vi "Project Data InitialS3.vi"(11 "configuration file path":path=path "C:/Users/MyUser/Desktop/新文字文件 - 複製.txt") -> (1 "Step Content":string[][](table), 2 "Retry":i32, 3 "process cluster":cluster{string[], i32[]})   [LabVIEW 2019]
uses:
  <vilib>/Utility/config.llb/Read Key (String).vi
  <vilib>/Utility/config.llb/NI_LVConfig.lvlib
  Ctrl/StationCmdSelect.ctl
  FlowCtrl Class/LineScan/LineScan.lvclass
  Ctrl/MeasureDisplayTab.ctl
  LLB/Commonly VI/Main Glb.vi
  LLB/Commonly VI.lvlib
  Ctrl/Table Save.ctl
  Ctrl/Auto Inspection Station Name2.ctl
  Ctrl/Auto Inspection Data Name.ctl
  Ctrl/S2 Station IO.ctl
panel:
  out "S2 receive":string
  out "Blue Scan2 receive":string
  out "T2 buffer":string
  out "T2 μA":dbl format="%#_6f"
  out "T1 buffer":string
  out "T1 μA":dbl format="%#_6f"
  in  "error in (no error)":errorcluster
  out "Blue Scan receive":string
  out "S1 receive":string
  out "Program receive":string
  out "Initial receive":string
  out "Act Step":i32
  out "retry次數":string[](array[string])
  in  "stop":bool
  out "Boolean":bool=TRUE
  in  "Numeric 3":i32
  out "format receive":string
  out "CurrentCmd":string
  out "Numeric":dbl
  out "LOG":string[][](array[string])
  in  "Enum":T1(ring)=enum."Add"
  in  "Table Control 3":string[][](table)=[["PCBA BARCODE", ""], ["硬體(Tool初始化)", ""], ["company(Tool初始化)", ""], ["耗電流 uA(電流表)", "T"], ["電池負載電壓", "T"], ["晶片ID(Tool FORMAT)", "F"], ["雷雕ID(TOOl scan、藍芽接收器)", "S"], ["Format(Tool FORMAT)", "F"], ["Programe(Tool Programe)", "P"]]
  in  "SN":string
  out "Array 3":cluster{"Table Control":string[][]}[](array[cluster])
  in  "Table Control":string[][](table)=[["PCBA BARCODE", ""], ["硬體(Tool初始化)", ""], ["company(Tool初始化)", ""], ["耗電流 uA(電流表)", "T"], ["電池負載電壓", "T"], ["晶片ID(Tool FORMAT)", "F"], ["雷雕ID(TOOl scan、藍芽接收器)", "S"], ["Format(Tool FORMAT)", "F"], ["Programe(Tool Programe)", "P"]]
  out "subarray":string[](array[string])
  out "array":string[](array[string])
  out "Process":string[](array[string])
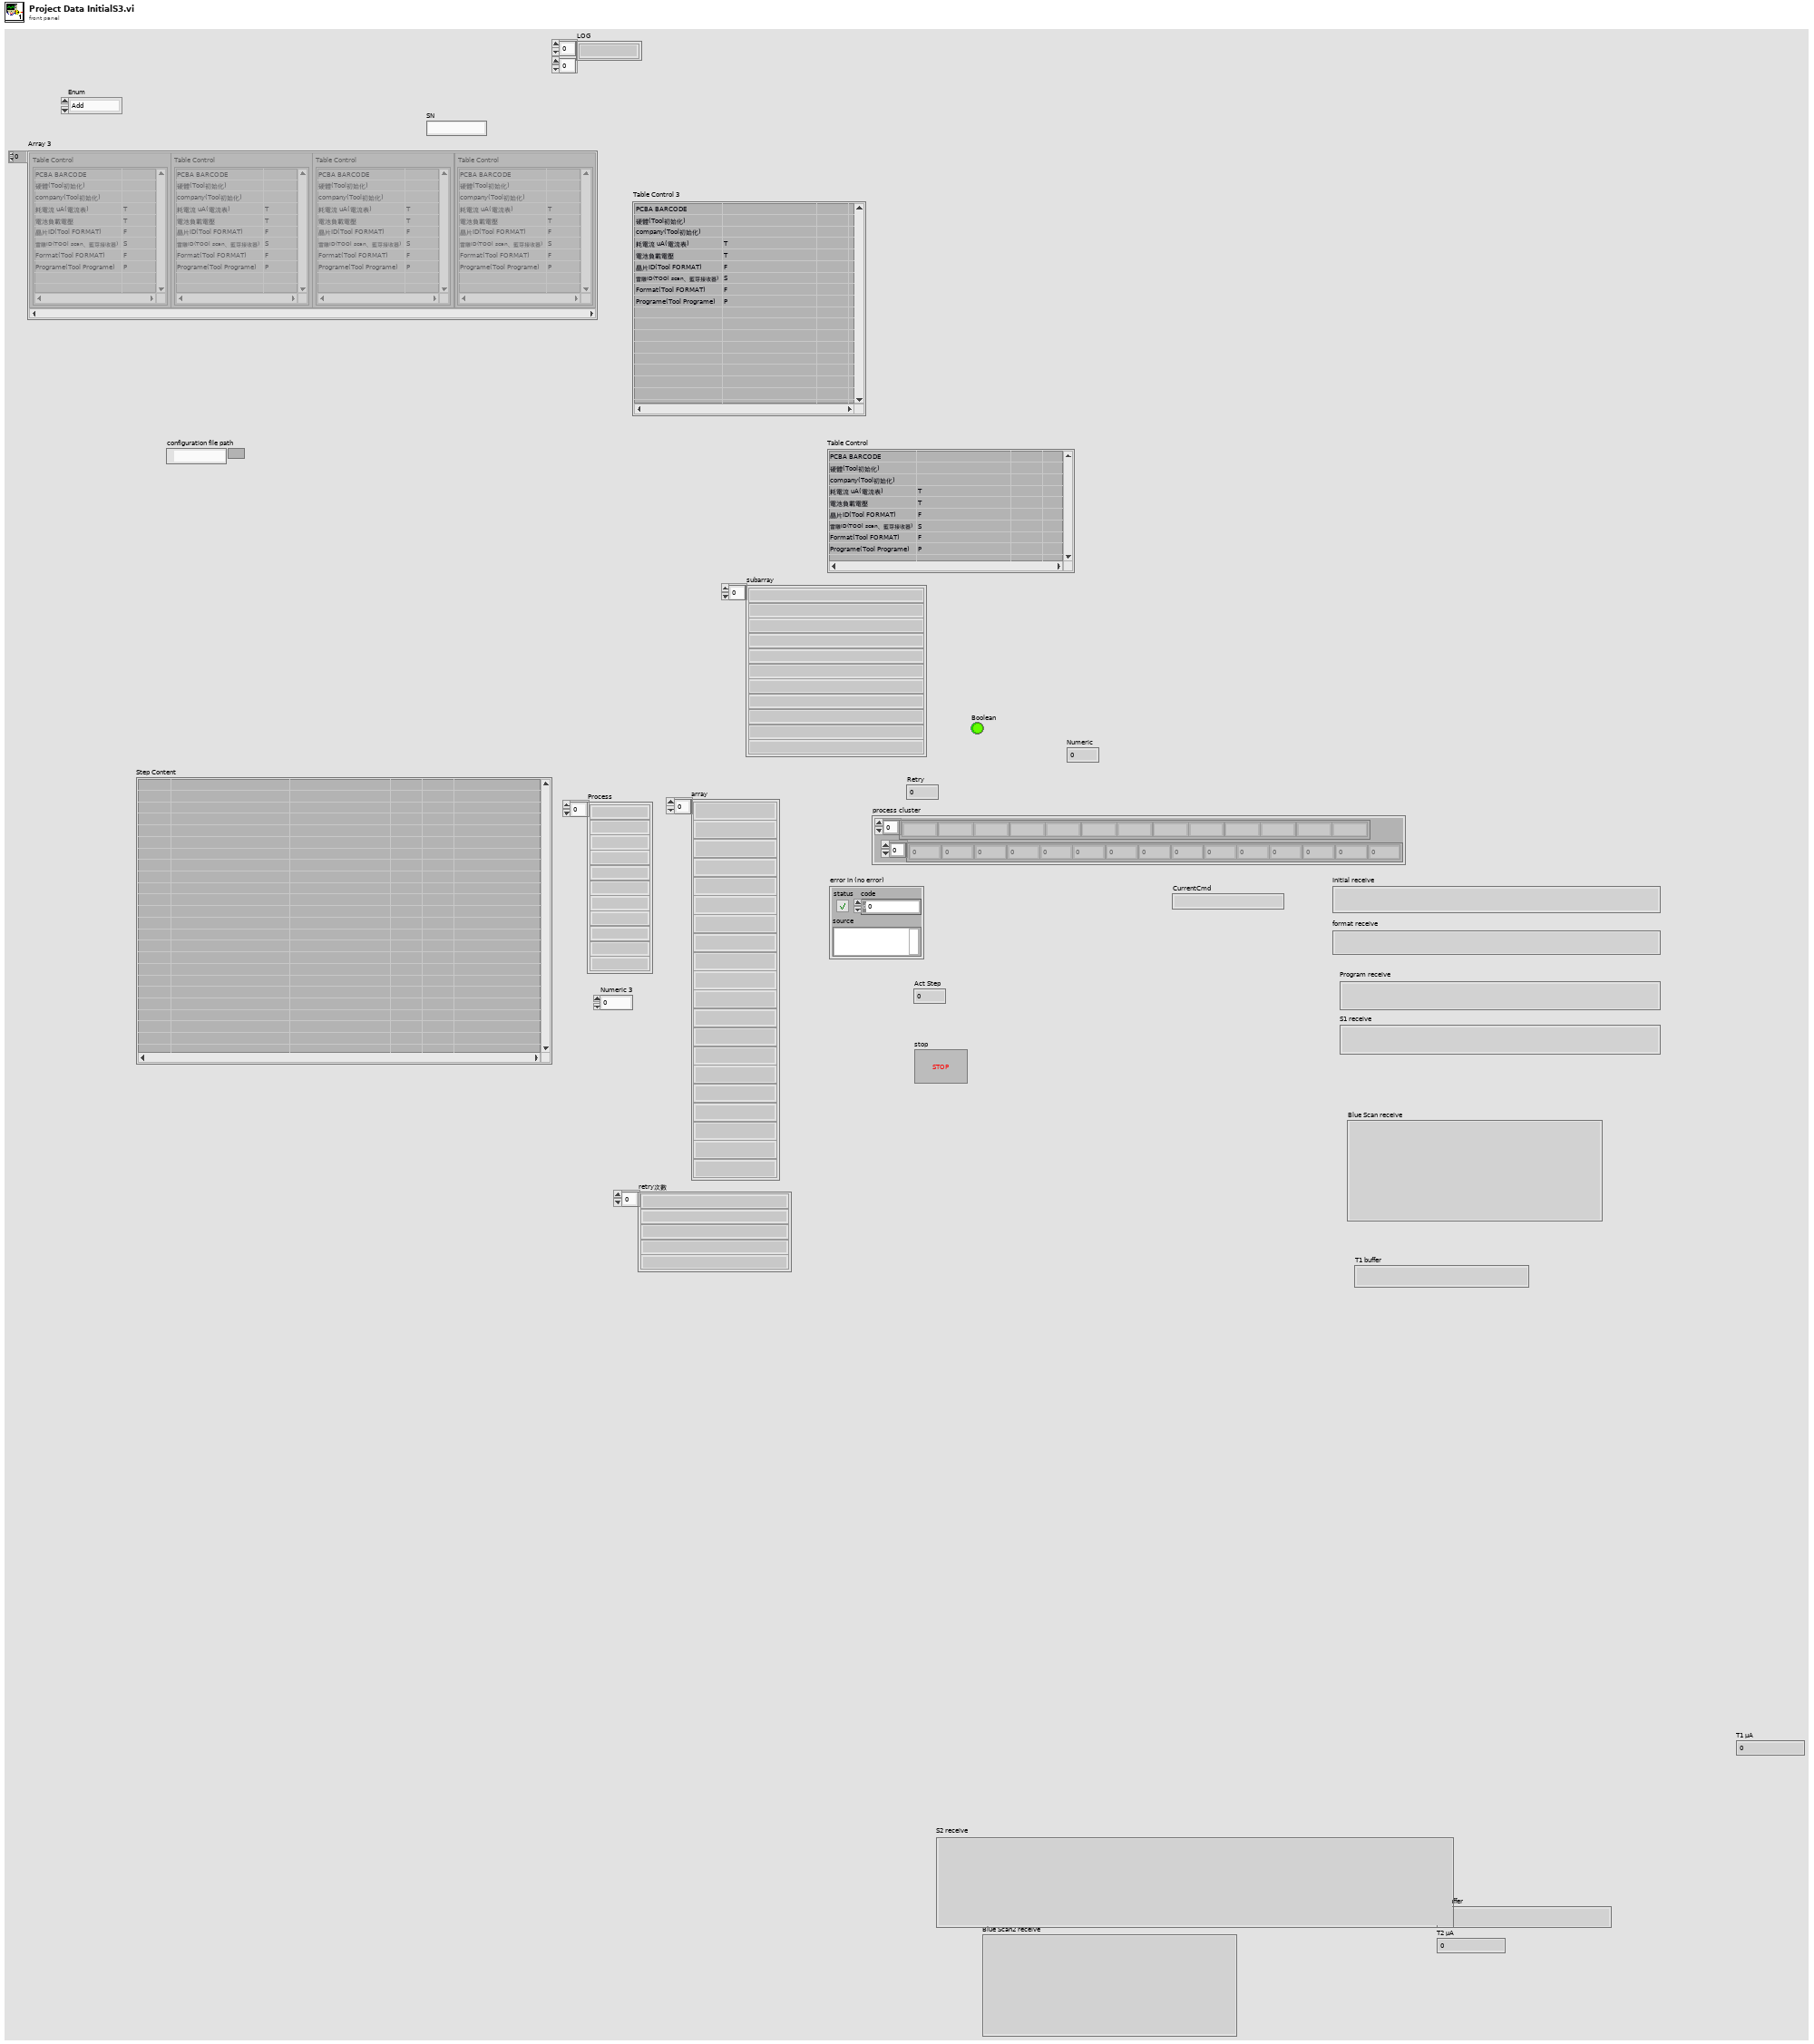
[diagram p1: front panel]
types:
  T1 = enum16{"initial", "Add", "Write", "Replace", "Delete", "REad"}
  T2 = typedef "NI_LVConfig.lvlib/Config Data RefNum.ctl" = refnum<k1>
  T3 = typedef "StationCmdSelect.ctl" = enum16{"Action", "Command", "Return", "DTime", "Retry"}
  T4 = typedef "Auto Inspection Data Name.ctl" = enum16{"LocalRun", "ItemSN(TimeCode)", "CurrentAction", "Error", "Data", "OKNG", "電壓值", "電壓值判斷", "電流值", "電流值判斷", "Laser1 Data", "Laser2 Data", "Laser OKNG", "StationNO"}
  T5 = typedef "Auto Inspection Station Name2.ctl" = enum16{"S1Barcode", "S2Measure", "S3Measure", "S4Measure", "S5Measure", "S11_LaserCheck", "S8_Vision AI"}
  T6 = typedef "Table Save.ctl" = enum16{"initial", "Add", "Write", "Replace", "Delete", "REad", "RedTable", "Load"}
  T7 = typedef "MeasureDisplayTab.ctl" = enum16{"Tray Barcode", "PCBA BARCODE", "硬體(Tool初始化)", "company(Tool初始化)", "耗電流 uA(電流表)", "電池負載電壓", "晶片ID(Tool FORMAT)", "雷雕ID(TOOl scan、藍芽接收器)", "Format(Tool FORMAT)", "Programe(Tool Programe)", "MAC(藍芽接收器)", "ID(藍芽接收器)", "KPA(藍芽接收器)", "溫度(藍芽接收器)", "SENSOR電池電壓(藍芽接收器)", "RSSI(藍芽接收器)", "SensorType_315(FSK scan)", "FSKsnVol_315(FSK scan)", "FSKscanl_315(FSK scan)", "P_315(FSK scan)", "T_315(FSK scan)", "SensorType_433(ASK scan)", "ASKsnVol_433(ASK scan)", "ASKscan_433(ASK scan)", "P_433(ASK scan)", "T_433(ASK scan)", "測高Data"}
  T8 = typedef "S2 Station IO.ctl" = enum16{"S2站PC動作中_20", "電流量測完成產品OK_21", "電流量測完成產品NG_22", "S2站Format 執行_23", "S2 Format OK_24", "S2 Format NG_25", "S2站燒入執行_26", "S2站燒入OK_27", "S2站燒入NG_28", "S2站動作完成_29", "S3 PC動作中_30", "S3 Format 此站執行_31", "S3 Format OK_32", "S3 Format NG_33", "S3 燒入程式 此站執行_34", "S3 燒入程式 OK_35", "S3 燒入程式 NG_36", "S3 備用_37", "S3 備用_38", "S3 動作完成_39", "S4 PC動作中_40", "S4 量測完成 產品正常_41", "S4 量測完成 產品NG_42", "S4 Format 此站執行_43", "S4 Format OK_44", "S4 Format NG_45", "S4 燒入 此站不執行_46", "S4 燒入程式 OK_47", "S4 燒入程式 NG_48", "S4 藍芽Scan OK_49", "S4 藍芽Scan NG_50", "S4 動作完成_51", "給PLC要量電流訊號", "給PLC要量電壓訊號"}
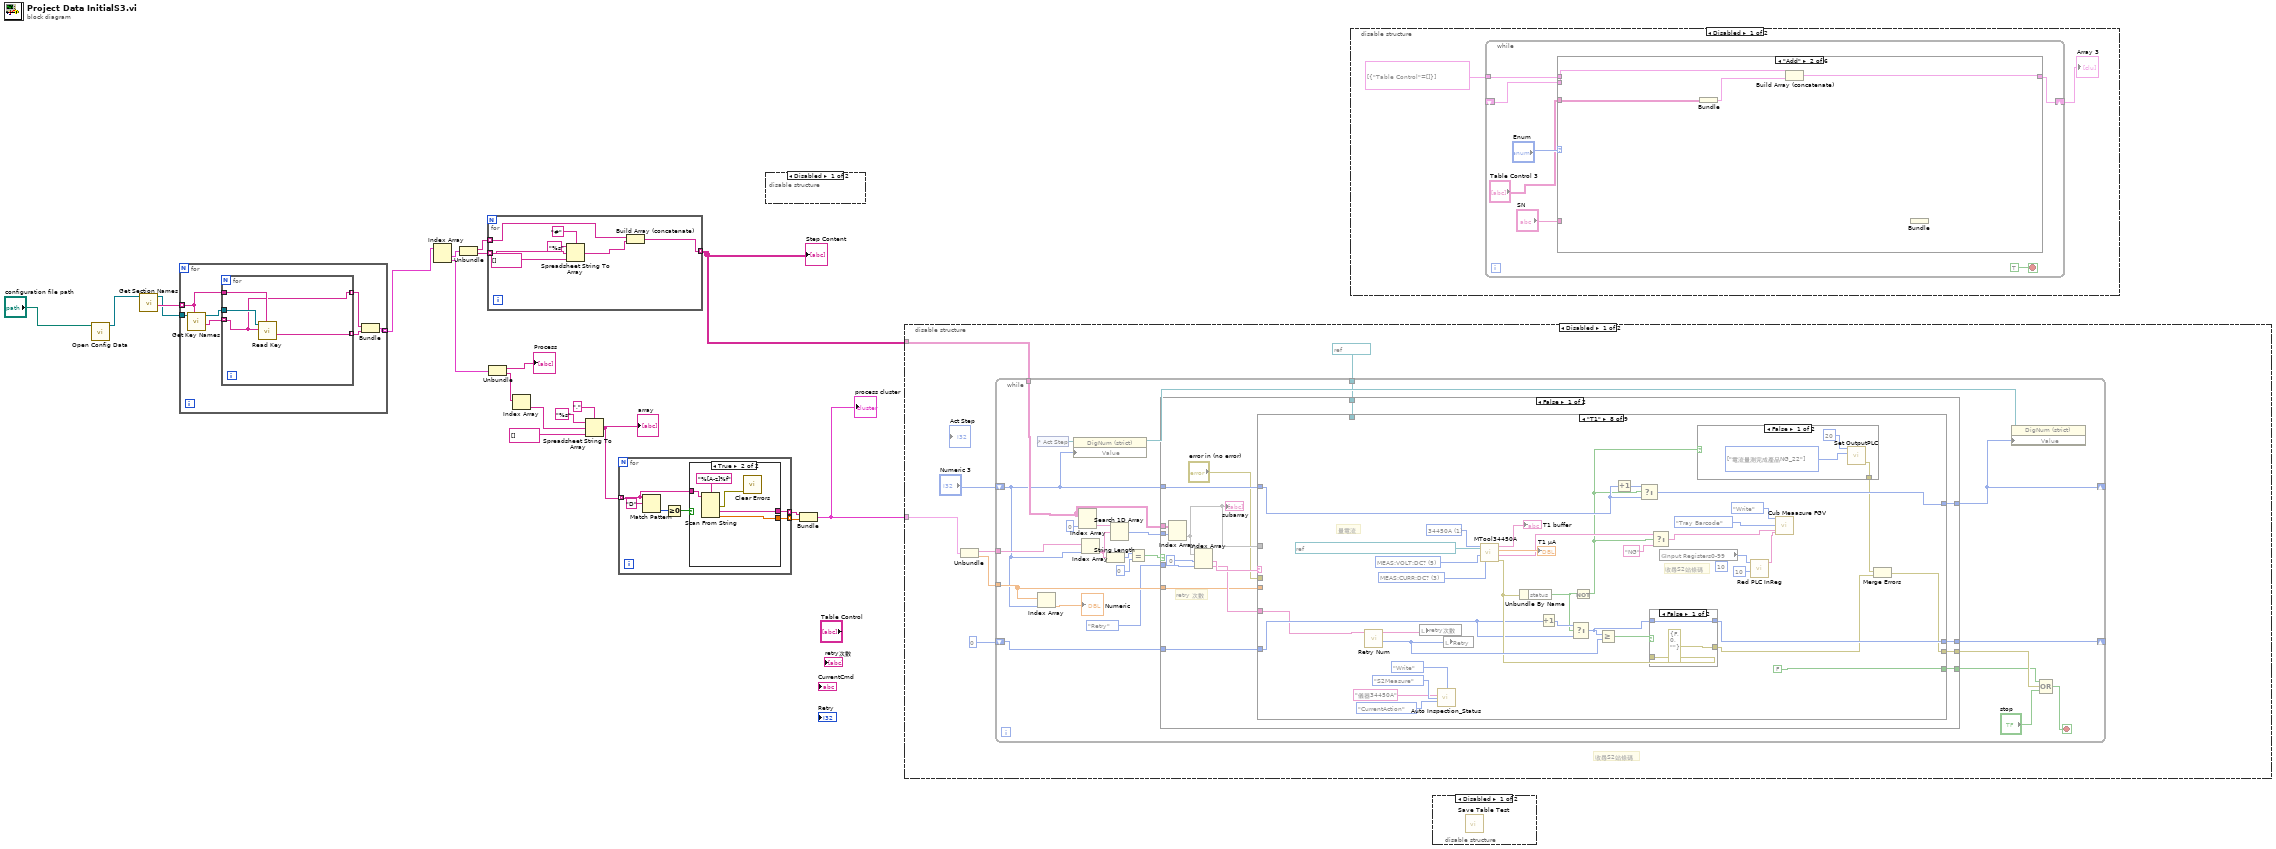
[diagram p0: block diagram]
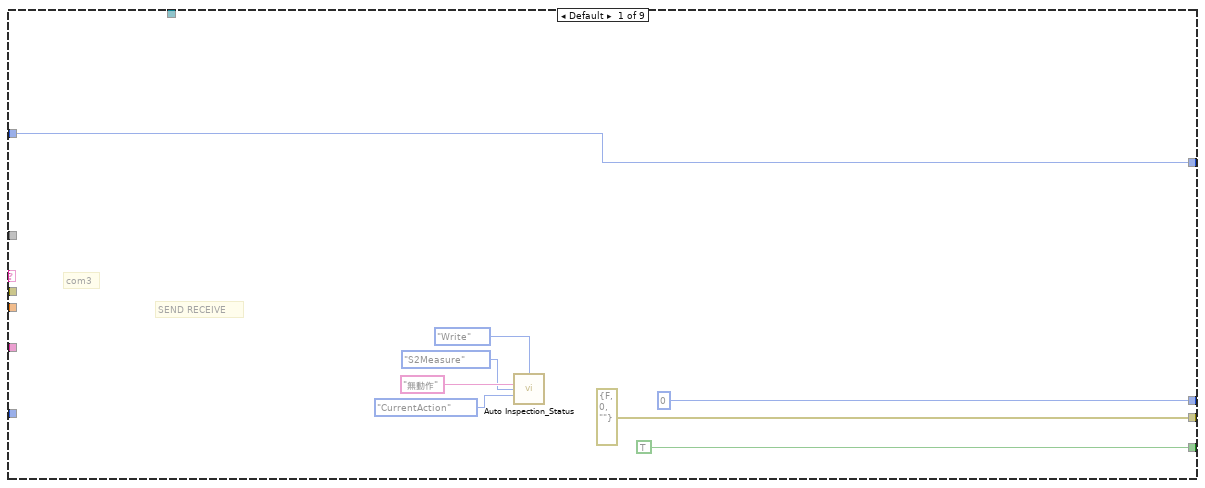
[diagram p3: hidden frame]
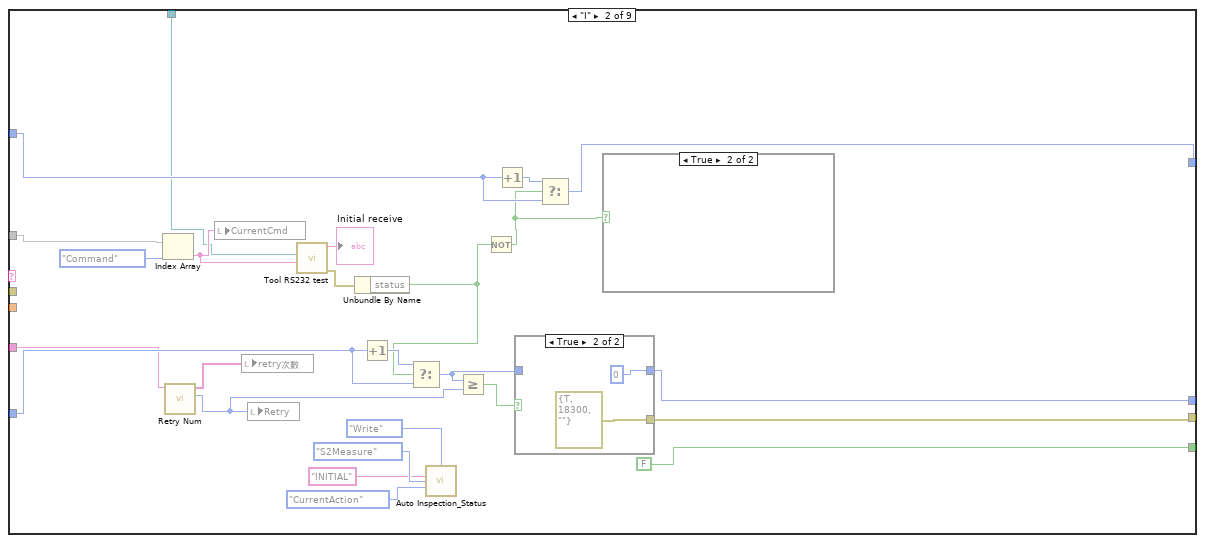
[diagram p4: hidden frame]
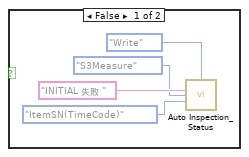
[diagram p5: hidden frame]
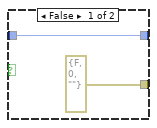
[diagram p6: hidden frame]
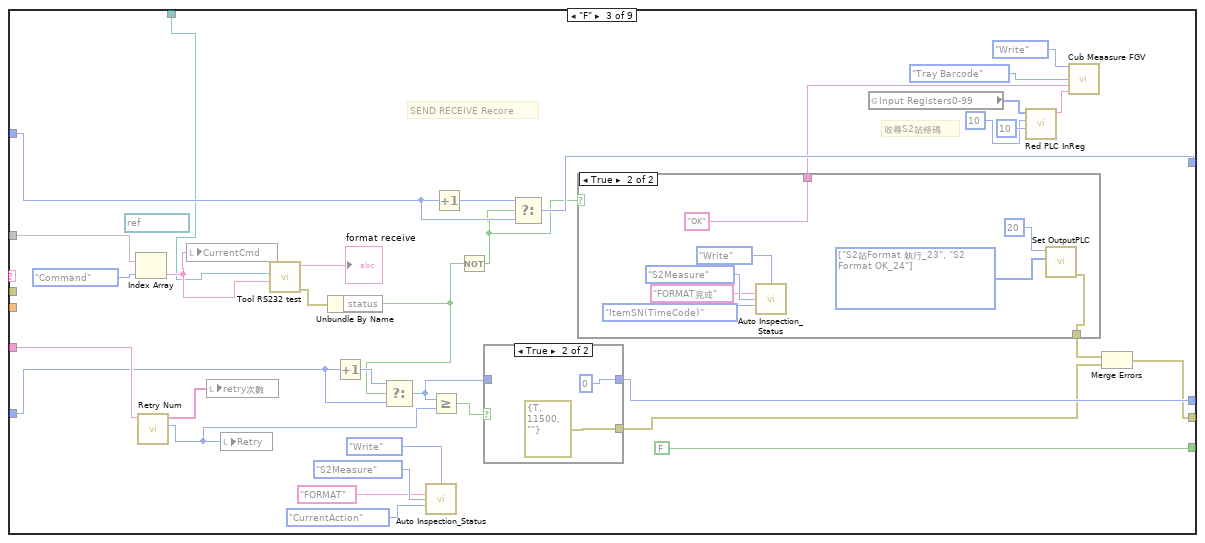
[diagram p7: hidden frame]
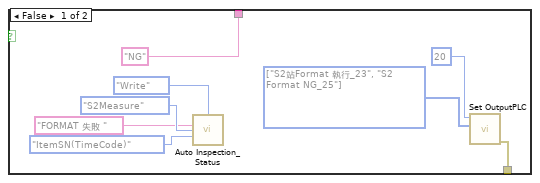
[diagram p8: hidden frame]
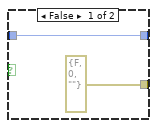
[diagram p9: hidden frame]
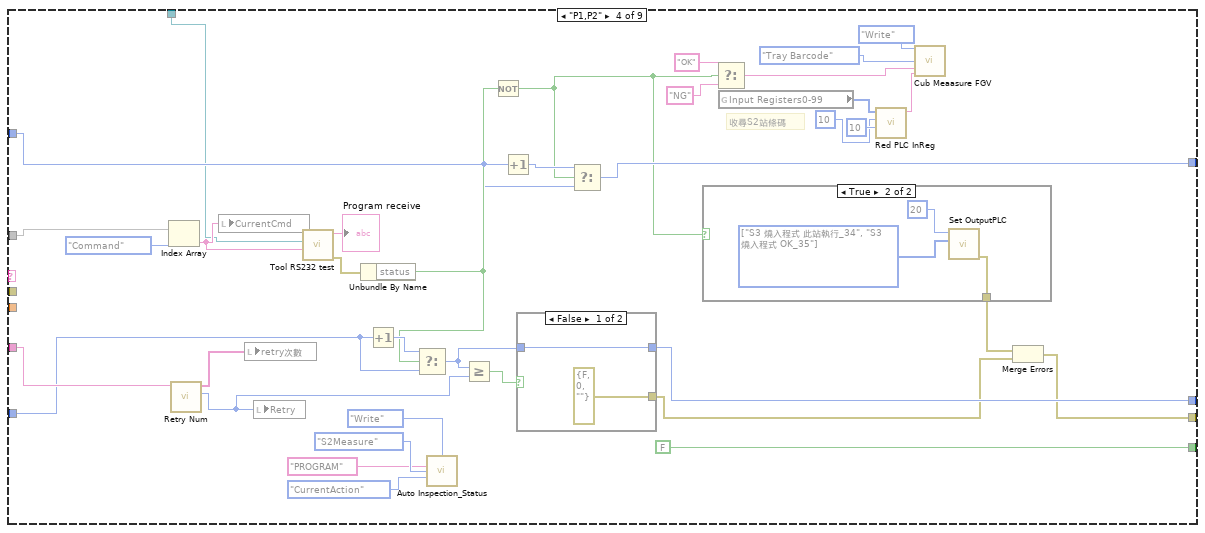
[diagram p10: hidden frame]
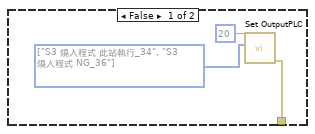
[diagram p11: hidden frame]
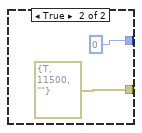
[diagram p12: hidden frame]
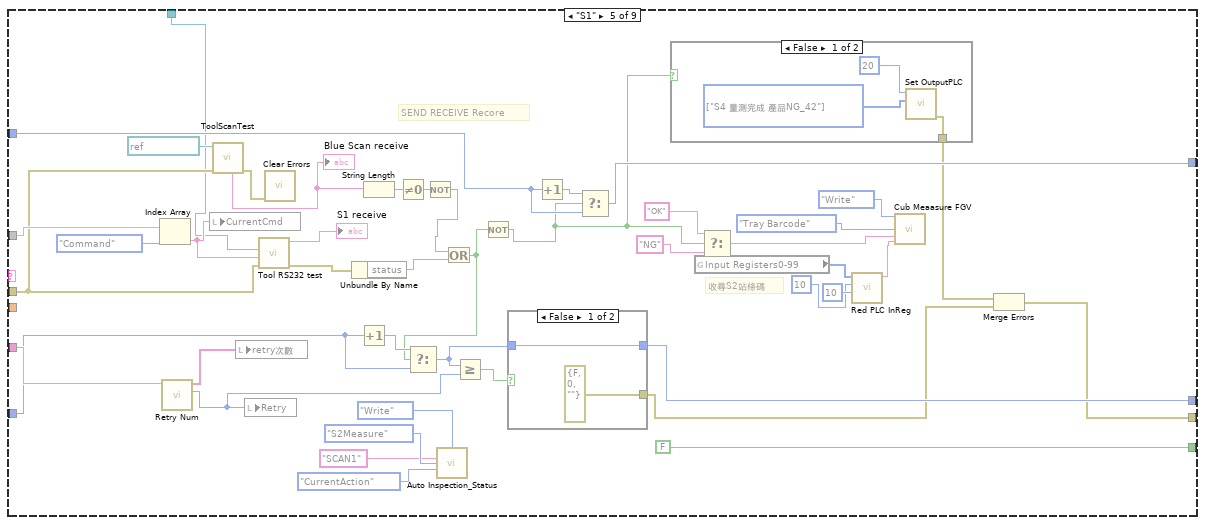
[diagram p13: hidden frame]
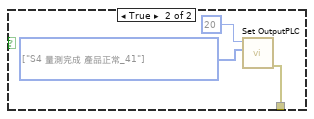
[diagram p14: hidden frame]
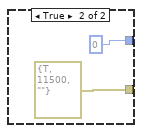
[diagram p15: hidden frame]
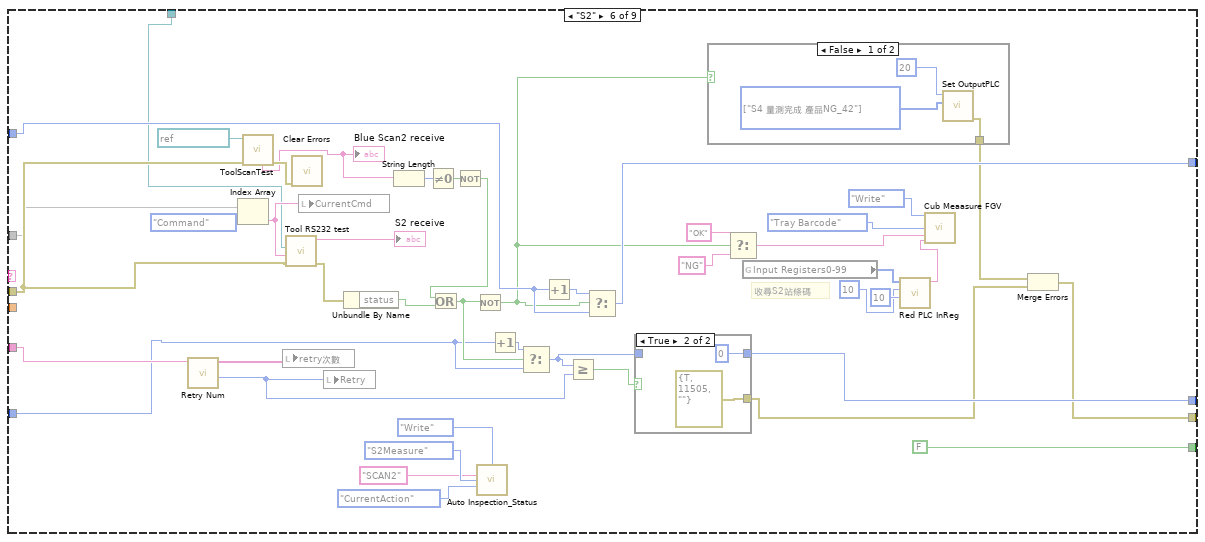
[diagram p16: hidden frame]
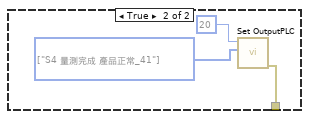
[diagram p17: hidden frame]
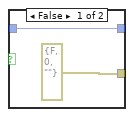
[diagram p18: hidden frame]
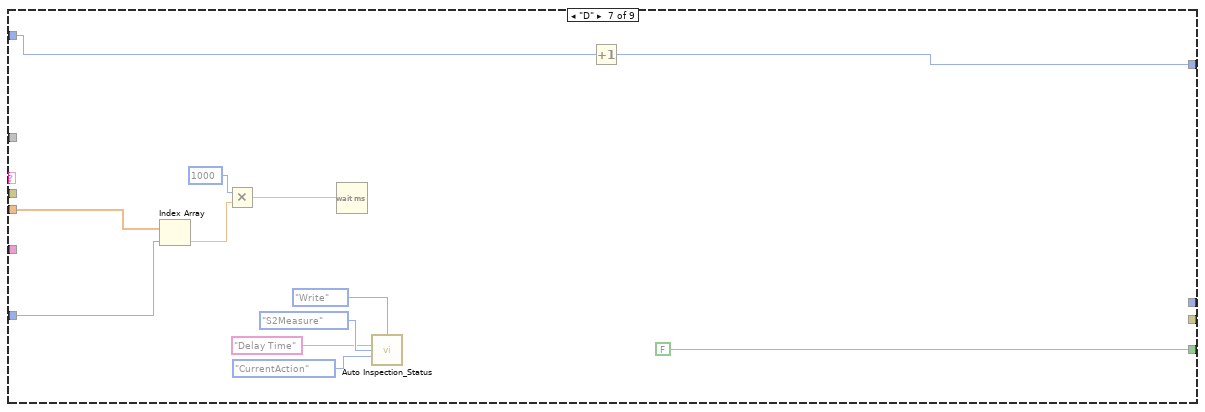
[diagram p19: hidden frame]
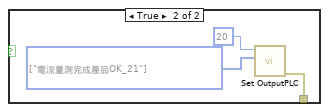
[diagram p20: hidden frame]
diagram:
  n1 = call <vilib>:"Open Config Data.vi"("configuration file path"="configuration file path") -> ("refnum"=w19:T2)  [unwired: 8 in, 2 out]
  n2 = call <vilib>:"Get Section Names.vi"("refnum"=w19) -> ("section names"=w18:string[], "refnum out"=w17:T2)  [unwired: 8 in, 1 out]
  n3 = for {
    tunnel: w17 -> [w27]
    tunnel: w18 -> [w22] mode=indexing
    tunnel: [w24] -> w15 mode=indexing
    n4 = call <vilib>:"Get Key Names.vi"("section"=w22, "refnum"=w27) -> ("key names"=w26:string[], "refnum out"=w23:T2)  [unwired: 6 in, 2 out]
    n5 = for {
      tunnel: w26 -> [w28] mode=indexing
      tunnel: [w31] -> w25 mode=indexing
      tunnel: w23 -> [w30]
      tunnel: w22 -> [w29]
      tunnel: [w28] -> w21 mode=indexing
      n6 = call-poly <vilib>:"Read Key.vi"("section"=w29, "key"=w28, "refnum"=w30) -> ("value"=w31:string)  [unwired: 5 in, 3 out]
    }
    n7 = Bundle(w21, w25) -> (w24:cluster{string[], string[]})  [unwired: 1 in]
  }
  n8 = Index Array(array=w15) -> (element #1=w11:cluster{string[], string[]}, element #2=w14:cluster{string[], string[]})  [unwired: 2 in]
  n9 = Unbundle(w11) -> (w12:string[], w13:string[])
  n10 = for {
    tunnel: w13 -> [w36] mode=indexing
    tunnel: [w32] -> w2 mode=indexing
    tunnel: w12 -> [w33] mode=indexing
    n11 = Spreadsheet String To Array(delimiter (Tab)="#", format string="%s", spreadsheet string=w36, array type (2D Dbl)=string[] []) -> (array=w34:string[])
    n12 = Build Array (concatenate)(w33, w34) -> (w32:string[])
  }
  "Step Content" <- w2
  n13 = Unbundle(w14) -> (→"Process":string[], w7:string[])
  n14 = Index Array(array=w7) -> (element=w6:string)  [unwired: 1 in]
  n15 = Spreadsheet String To Array(delimiter (Tab)=",", format string="%s", spreadsheet string=w6, array type (2D Dbl)=string[] []) -> (array=w5:string[])
  "array" <- w5
  n16 = for {
    tunnel: w5 -> [w39] mode=indexing
    tunnel: [w44] -> w4 mode=indexing
    tunnel: [w43] -> w3 mode=indexing
    n17 = Match Pattern(string=w39, regular expression="D") -> (offset past match=w41:i32)  [unwired: 1 in, 3 out]
    n18 = Greater Or Equal To 0?(x=w41) -> (x >= 0?=w40:bool)
    n19 = case shown="True" w40 {
      tunnel: [w46 w50] -> w44
      tunnel: [-1.0 w49] -> w43
      tunnel: w39 -> [w46 w47]
      frame False {
      }
      frame True {
        n20 = Scan From String(format string="%[A-z]%f", input string=w47) -> (error out=w48:errorcluster, output 1=w50:string, output 2=w49:dbl)  [unwired: 4 in, 2 out]
        n21 = call <vilib>:"Clear Errors.vi"("error in (no error)"=w48) -> ()  [unwired: 5 in, 2 out]
      }
    }
  }
  n22 = disable-structure shown="Disabled" {
    frame Disabled {
    }
    frame Enabled {
    }
  }
  n23 = Bundle(w4, w3) -> (w1:cluster{string[], dbl[]})  [unwired: 1 in]
  "process cluster" <- w1
  n24 = disable-structure shown="Disabled" {
    disable-tunnel: w2 -> [w56 _]
    disable-tunnel: w1 -> [w55 _]
    frame Disabled {
      # "收尋S2站條碼"
      n25 = Unbundle(w55) -> (w58:string[], w57:dbl[])
      n26 = while {
        tunnel: w58 -> [w81]
        tunnel: w57 -> [w80]
        tunnel: w56 -> [w79]
        shift-right: [w62] -> _
        shift-left: 0 -> [w66]
        shift-right: [w63] -> _
        shift-left: "Numeric 3" -> [w60]
        tunnel: refnum<visa-resource-name> "COM2" ("VISA resource name") -> [w59]
        stop <- w67 stop-if-true
        n27 = control-ref of="Act Step"() -> (w65:refnum<vi>)
        n28 = Index Array(array=w80, index=w60) -> (element=→"Numeric":dbl)
        n29 = property class="DigNum (strict)"(reference=w65, "Value"=w60) -> (reference out=w64:refnum<vi>)  [unwired: 1 in, 1 out]
        n30 = Index Array(array=w79, index (col)=0 ("disabled index (col)")) -> (element=w77:string[])  [unwired: 1 in]
        n31 = Index Array(array=w81, index=w60) -> (element=w74:string)
        n32 = String Length(string=w74) -> (length=w73:i32)
        n33 = Search 1D Array(1D array=w77, element=w74) -> (index of element=w76:i32)  [unwired: 1 in]
        n34 = Equal?(x=w73, y=0) -> (x = y?=w71:bool)
        n35 = case shown="False" w71 {
          tunnel: w79 -> [w97 _]
          tunnel: w76 -> [w96 _]
          tunnel: w80 -> [w92 _]
          tunnel: w66 -> [w90 _]
          tunnel: StationCmdSelect."Retry" -> [w89 _]
          tunnel: [w88 _] -> w68
          tunnel: w60 -> [w87 _]
          tunnel: [w86 _] -> w63
          tunnel: [w85 _] -> w62
          tunnel: [w84 w451] -> w61
          tunnel: w59 -> [w82 _]
          frame False {
            # "retry 次數"
            n36 = Index Array(array=w97, index (row)=w96) -> (element=w91:string[])  [unwired: 1 in]
            "subarray" <- w91
            n37 = Index Array(array=w91, index #1=0 ("index"), index #2=w89) -> (element #1=w94:string, element #2=w93:string)
            n38 = case shown="\"T1\"" w94 {
              tunnel: w92 -> [_ _ _ _ _ _ w357 _ _]
              tunnel: w93 -> [_ w116 w169 w215 w271 w317 _ w378 w423]
              tunnel: w91 -> [_ w118 w172 w214 w268 w318 _ _ _]
              tunnel: w90 -> [_ w117 w166 w212 w266 w316 w354 w379 w424]
              tunnel: [errorcluster {"status"=FALSE, "code"=0, "source"=""} ("error constant") w121 w140 w194 w240 w294 _ w359 w405] -> w88
              tunnel: w87 -> [w105 w119 w161 w211 w270 w320 w352 w377 w425]
              tunnel: [w105 w115 w160 w217 w269 w313 w351 w376 w426] -> w86
              tunnel: [0 w120 w158 w216 w272 w315 _ w375 w428] -> w85
              tunnel: [TRUE FALSE FALSE FALSE FALSE FALSE FALSE FALSE FALSE] -> w84
              tunnel: "error in (no error)" -> [_ _ _ _ w263 w319 _ _ _]
              tunnel: w82 -> [_ w106 w139 w193 w239 w293 _ _ _]
              frame Default {
                # "SEND RECEIVE"
                # "com3"
                n39 = call "Auto Inspection_Status.vi"("Action"=enum16{"Initial", "Write", "Read"}."Write", "DataIn"="無動作", "Station"=Auto_Inspection_Station_Name2."S2Measure", "Data"=Auto_Inspection_Data_Name."CurrentAction") -> ()  [unwired: 9 in, 3 out]
              }
              frame "I" {
                n40 = Index Array(array=w118, index=StationCmdSelect."Command") -> (element=w113:string)
                n41 = call "Retry Num.vi"("String"=w116) -> ("Numeric"=w127:i32, "retry次數"=w114:string[])  [unwired: 9 in]
                n42 = local write "CurrentCmd"(w113) -> ()
                n43 = local write "retry次數"(w114) -> ()
                n44 = local write "Retry"(w127) -> ()
                n45 = call "Tool RS232 test.vi"("Cmd In"=w113, "VISA resource name"=w106) -> ("error out"=w128:errorcluster, "receive string"=→"Initial receive":string)  [unwired: 8 in]
                n46 = Unbundle By Name(w128) -> ("status"=w124:bool)
                n47 = Increment(x=w117) -> (x+1=w129:i32)
                n48 = Select(t=w129, s=w124, f=w117) -> (s? t:f=w123:i32)
                n49 = call "Auto Inspection_Status.vi"("Action"=enum16{"Initial", "Write", "Read"}."Write", "DataIn"="INITIAL", "Station"=Auto_Inspection_Station_Name2."S2Measure", "Data"=Auto_Inspection_Data_Name."CurrentAction") -> ()  [unwired: 9 in, 3 out]
                n50 = Greater Or Equal?(x=w123, y=w127) -> (x >= y?=w126:bool)
                n51 = Not(x=w124) -> (.not. x?=w107:bool)
                n52 = Increment(x=w119) -> (x+1=w125:i32)
                n53 = case shown="True" w126 {
                  tunnel: [errorcluster {"status"=FALSE, "code"=0, "source"=""} ("error constant") errorcluster {"status"=TRUE, "code"=18300, "source"=""} ("error constant")] -> w121
                  tunnel: w123 -> [w135 _]
                  tunnel: [w135 0] -> w120
                  frame False {
                  }
                  frame True {
                  }
                }
                n54 = Select(t=w125, s=w107, f=w119) -> (s? t:f=w115:i32)
                n55 = case shown="True" w107 {
                  frame False {
                    n56 = call "Auto Inspection_Status.vi"("Action"=enum16{"Initial", "Write", "Read"}."Write", "DataIn"="INITIAL 失敗 ", "Station"=Auto_Inspection_Station_Name2."S3Measure", "Data"=Auto_Inspection_Data_Name."ItemSN(TimeCode)") -> ()  [unwired: 9 in, 3 out]
                  }
                  frame True {
                  }
                }
              }
              frame "F" {
                (unwired) refnum<visa-resource-name> "COM8" ("VISA resource name")
                # "收尋S2站條碼"
                # "SEND RECEIVE Recore"
                n57 = Index Array(array=w172, index=StationCmdSelect."Command") -> (element=w157:string)
                n58 = call "Retry Num.vi"("String"=w169) -> ("Numeric"=w165:i32, "retry次數"=w156:string[])  [unwired: 9 in]
                n59 = local write "CurrentCmd"(w157) -> ()
                n60 = local write "retry次數"(w156) -> ()
                n61 = local write "Retry"(w165) -> ()
                n62 = call "Tool RS232 test.vi"("Cmd In"=w157, "VISA resource name"=w139) -> ("error out"=w167:errorcluster, "receive string"=→"format receive":string)  [unwired: 8 in]
                n63 = Unbundle By Name(w167) -> ("status"=w162:bool)
                n64 = Increment(x=w166) -> (x+1=w168:i32)
                n65 = Select(t=w168, s=w162, f=w166) -> (s? t:f=w159:i32)
                n66 = call "Auto Inspection_Status.vi"("Action"=enum16{"Initial", "Write", "Read"}."Write", "DataIn"="FORMAT", "Station"=Auto_Inspection_Station_Name2."S2Measure", "Data"=Auto_Inspection_Data_Name."CurrentAction") -> ()  [unwired: 9 in, 3 out]
                n67 = Greater Or Equal?(x=w159, y=w165) -> (x >= y?=w164:bool)
                n68 = Increment(x=w161) -> (x+1=w163:i32)
                n69 = Not(x=w162) -> (.not. x?=w154:bool)
                n70 = case shown="True" w164 {
                  tunnel: [errorcluster {"status"=FALSE, "code"=0, "source"=""} ("error constant") errorcluster {"status"=TRUE, "code"=11500, "source"=""} ("error constant")] -> w141
                  tunnel: w159 -> [w189 _]
                  tunnel: [w189 0] -> w158
                  frame False {
                  }
                  frame True {
                  }
                }
                n71 = Select(t=w163, s=w154, f=w161) -> (s? t:f=w160:i32)
                n72 = case shown="True" w154 {
                  tunnel: ["NG" "OK"] -> w147
                  tunnel: [w173 w181] -> w142
                  frame False {
                    w175 = T8[] [enum."S2站Format 執行_23", enum."S2 Format NG_25"] items=["S2站PC動作中_20", "電流量測完成產品OK_21", "電流量測完成產品NG_22", "S2站Format 執行_23", "S2 Format OK_24", "S2 Format NG_25", "S2站燒入執行_26", "S2站燒入OK_27", "S2站燒入NG_28", "S2站動作完成_29", "S3 PC動作中_30", "S3 Format 此站執行_31", "S3 Format OK_32", "S3 Format NG_33", "S3 燒入程式 此站執行_34", "S3 燒入程式 OK_35", "S3 燒入程式 NG_36", "S3 備用_37", "S3 備用_38", "S3 動作完成_39", "S4 PC動作中_40", "S4 量測完成 產品正常_41", "S4 量測完成 產品NG_42", "S4 Format 此站執行_43", "S4 Format OK_44", "S4 Format NG_45", "S4 燒入 此站不執行_46", "S4 燒入程式 OK_47", "S4 燒入程式 NG_48", "S4 藍芽Scan OK_49", "S4 藍芽Scan NG_50", "S4 動作完成_51", "給PLC要量電流訊號", "給PLC要量電壓訊號"]
                    n73 = call "Auto Inspection_Status.vi"("Action"=enum16{"Initial", "Write", "Read"}."Write", "DataIn"="FORMAT 失敗 ", "Station"=Auto_Inspection_Station_Name2."S2Measure", "Data"=Auto_Inspection_Data_Name."ItemSN(TimeCode)") -> ()  [unwired: 9 in, 3 out]
                    n74 = call "Set OutputPLC.vi"("Array"=w175, "Address In"=20) -> ("Error Out"=w173:errorcluster[])  [unwired: 9 in]
                  }
                  frame True {
                    w183 = T8[] [enum."S2站Format 執行_23", enum."S2 Format OK_24"] items=["S2站PC動作中_20", "電流量測完成產品OK_21", "電流量測完成產品NG_22", "S2站Format 執行_23", "S2 Format OK_24", "S2 Format NG_25", "S2站燒入執行_26", "S2站燒入OK_27", "S2站燒入NG_28", "S2站動作完成_29", "S3 PC動作中_30", "S3 Format 此站執行_31", "S3 Format OK_32", "S3 Format NG_33", "S3 燒入程式 此站執行_34", "S3 燒入程式 OK_35", "S3 燒入程式 NG_36", "S3 備用_37", "S3 備用_38", "S3 動作完成_39", "S4 PC動作中_40", "S4 量測完成 產品正常_41", "S4 量測完成 產品NG_42", "S4 Format 此站執行_43", "S4 Format OK_44", "S4 Format NG_45", "S4 燒入 此站不執行_46", "S4 燒入程式 OK_47", "S4 燒入程式 NG_48", "S4 藍芽Scan OK_49", "S4 藍芽Scan NG_50", "S4 動作完成_51", "給PLC要量電流訊號", "給PLC要量電壓訊號"]
                    n75 = call "Auto Inspection_Status.vi"("Action"=enum16{"Initial", "Write", "Read"}."Write", "DataIn"="FORMAT完成", "Station"=Auto_Inspection_Station_Name2."S2Measure", "Data"=Auto_Inspection_Data_Name."ItemSN(TimeCode)") -> ()  [unwired: 9 in, 3 out]
                    n76 = call "Set OutputPLC.vi"("Array"=w183, "Address In"=20) -> ("Error Out"=w181:errorcluster[])  [unwired: 9 in]
                  }
                }
                n77 = global read "Main Glb.vi" "Input Registers0-99"() -> (w146:u16[])
                n78 = call "Red PLC InReg.vi"("length"=10, "index"=10, "Input Registers Arr"=w146) -> ("Rad In Reg"=w143:string)  [unwired: 7 in, 1 out]
                n79 = call "Cub Meaasure FGV.vi"("Action"=Table_Save."Write" ("Enum"), 7:MeasureDisplayTab."Tray Barcode", "DataIn"=w147, "SN"=w143) -> ()  [unwired: 5 in, 7 out]
                n80 = Merge Errors(w142, w141) -> (w140:errorcluster)
              }
              frame "P1,P2" {
                # "收尋S2站條碼"
                n81 = Index Array(array=w214, index=StationCmdSelect."Command") -> (element=w228:string)
                n82 = call "Retry Num.vi"("String"=w215) -> ("Numeric"=w223:i32, "retry次數"=w227:string[])  [unwired: 9 in]
                n83 = local write "CurrentCmd"(w228) -> ()
                n84 = local write "retry次數"(w227) -> ()
                n85 = local write "Retry"(w223) -> ()
                n86 = call "Tool RS232 test.vi"("Cmd In"=w228, "VISA resource name"=w193) -> ("error out"=w224:errorcluster, "receive string"=→"Program receive":string)  [unwired: 8 in]
                n87 = Unbundle By Name(w224) -> ("status"=w220:bool)
                n88 = Increment(x=w212) -> (x+1=w225:i32)
                n89 = Select(t=w225, s=w220, f=w212) -> (s? t:f=w219:i32)
                n90 = call "Auto Inspection_Status.vi"("Action"=enum16{"Initial", "Write", "Read"}."Write", "DataIn"="PROGRAM", "Station"=Auto_Inspection_Station_Name2."S2Measure", "Data"=Auto_Inspection_Data_Name."CurrentAction") -> ()  [unwired: 9 in, 3 out]
                n91 = Greater Or Equal?(x=w219, y=w223) -> (x >= y?=w222:bool)
                n92 = Not(x=w220) -> (.not. x?=w197:bool)
                n93 = Increment(x=w211) -> (x+1=w221:i32)
                n94 = case shown="False" w222 {
                  tunnel: [errorcluster {"status"=FALSE, "code"=0, "source"=""} ("error constant") errorcluster {"status"=TRUE, "code"=11500, "source"=""} ("error constant")] -> w196
                  tunnel: w219 -> [w235 _]
                  tunnel: [w235 0] -> w216
                  frame False {
                  }
                  frame True {
                  }
                }
                n95 = Select(t=w221, s=w197, f=w211) -> (s? t:f=w217:i32)
                n96 = case shown="True" w197 {
                  tunnel: [w229 w232] -> w195
                  frame False {
                    w231 = T8[] [enum."S3 燒入程式 此站執行_34", enum."S3 燒入程式 NG_36"] items=["S2站PC動作中_20", "電流量測完成產品OK_21", "電流量測完成產品NG_22", "S2站Format 執行_23", "S2 Format OK_24", "S2 Format NG_25", "S2站燒入執行_26", "S2站燒入OK_27", "S2站燒入NG_28", "S2站動作完成_29", "S3 PC動作中_30", "S3 Format 此站執行_31", "S3 Format OK_32", "S3 Format NG_33", "S3 燒入程式 此站執行_34", "S3 燒入程式 OK_35", "S3 燒入程式 NG_36", "S3 備用_37", "S3 備用_38", "S3 動作完成_39", "S4 PC動作中_40", "S4 量測完成 產品正常_41", "S4 量測完成 產品NG_42", "S4 Format 此站執行_43", "S4 Format OK_44", "S4 Format NG_45", "S4 燒入 此站不執行_46", "S4 燒入程式 OK_47", "S4 燒入程式 NG_48", "S4 藍芽Scan OK_49", "S4 藍芽Scan NG_50", "S4 動作完成_51", "給PLC要量電流訊號", "給PLC要量電壓訊號"]
                    n97 = call "Set OutputPLC.vi"("Array"=w231, "Address In"=20) -> ("Error Out"=w229:errorcluster[])  [unwired: 9 in]
                  }
                  frame True {
                    w233 = T8[] [enum."S3 燒入程式 此站執行_34", enum."S3 燒入程式 OK_35"] items=["S2站PC動作中_20", "電流量測完成產品OK_21", "電流量測完成產品NG_22", "S2站Format 執行_23", "S2 Format OK_24", "S2 Format NG_25", "S2站燒入執行_26", "S2站燒入OK_27", "S2站燒入NG_28", "S2站動作完成_29", "S3 PC動作中_30", "S3 Format 此站執行_31", "S3 Format OK_32", "S3 Format NG_33", "S3 燒入程式 此站執行_34", "S3 燒入程式 OK_35", "S3 燒入程式 NG_36", "S3 備用_37", "S3 備用_38", "S3 動作完成_39", "S4 PC動作中_40", "S4 量測完成 產品正常_41", "S4 量測完成 產品NG_42", "S4 Format 此站執行_43", "S4 Format OK_44", "S4 Format NG_45", "S4 燒入 此站不執行_46", "S4 燒入程式 OK_47", "S4 燒入程式 NG_48", "S4 藍芽Scan OK_49", "S4 藍芽Scan NG_50", "S4 動作完成_51", "給PLC要量電流訊號", "給PLC要量電壓訊號"]
                    n98 = call "Set OutputPLC.vi"("Array"=w233, "Address In"=20) -> ("Error Out"=w232:errorcluster[])  [unwired: 9 in]
                  }
                }
                n99 = Select(t="OK" ("DataIn"), s=w197, f="NG" ("DataIn")) -> (s? t:f=w198:string)
                n100 = global read "Main Glb.vi" "Input Registers0-99"() -> (w206:u16[])
                n101 = call "Red PLC InReg.vi"("length"=10, "index"=10, "Input Registers Arr"=w206) -> ("Rad In Reg"=w205:string)  [unwired: 7 in, 1 out]
                n102 = call "Cub Meaasure FGV.vi"("Action"=Table_Save."Write" ("Enum"), 7:MeasureDisplayTab."Tray Barcode", "DataIn"=w198, "SN"=w205) -> ()  [unwired: 5 in, 7 out]
                n103 = Merge Errors(w195, w196) -> (w194:errorcluster)
              }
              frame "S1" {
                # "收尋S2站條碼"
                # "SEND RECEIVE Recore"
                n104 = Index Array(array=w268, index=StationCmdSelect."Command") -> (element=w281:string)
                n105 = call "Retry Num.vi"("String"=w271) -> ("Numeric"=w276:i32, "retry次數"=w280:string[])  [unwired: 9 in]
                n106 = local write "CurrentCmd"(w281) -> ()
                n107 = call "ToolScanTest.vi"("error in (no error)"=w263, "VISA resource name"=refnum<visa-resource-name> "COM10") -> ("error out"=w264:errorcluster, "read string 6"=w260:string)  [unwired: 4 in, 4 out]
                "Blue Scan receive" <- w260
                n108 = local write "retry次數"(w280) -> ()
                n109 = local write "Retry"(w276) -> ()
                n110 = call "Tool RS232 test.vi"("error in (no error)"=w263, "Cmd In"=w281, "VISA resource name"=w239) -> ("error out"=w277:errorcluster, "receive string"=→"S1 receive":string)  [unwired: 7 in]
                n111 = call <vilib>:"Clear Errors.vi"("error in (no error)"=w264) -> ()  [unwired: 5 in, 2 out]
                n112 = Unbundle By Name(w277) -> ("status"=w258:bool)
                n113 = Increment(x=w266) -> (x+1=w278:i32)
                n114 = String Length(string=w260) -> (length=w262:i32)
                n115 = Not Equal To 0?(x=w262) -> (x != 0?=w261:bool)
                n116 = Not(x=w261) -> (.not. x?=w259:bool)
                n117 = call "Auto Inspection_Status.vi"("Action"=enum16{"Initial", "Write", "Read"}."Write", "DataIn"="SCAN1", "Station"=Auto_Inspection_Station_Name2."S2Measure", "Data"=Auto_Inspection_Data_Name."CurrentAction") -> ()  [unwired: 9 in, 3 out]
                n118 = Or(x=w259, y=w258) -> (x .or. y?=w257:bool)
                n119 = Select(t=w278, s=w257, f=w266) -> (s? t:f=w273:i32)
                n120 = Greater Or Equal?(x=w273, y=w276) -> (x >= y?=w275:bool)
                n121 = Not(x=w257) -> (.not. x?=w243:bool)
                n122 = case shown="False" w275 {
                  tunnel: [errorcluster {"status"=FALSE, "code"=0, "source"=""} ("error constant") errorcluster {"status"=TRUE, "code"=11500, "source"=""} ("error constant")] -> w241
                  tunnel: w273 -> [w289 _]
                  tunnel: [w289 0] -> w272
                  frame False {
                  }
                  frame True {
                  }
                }
                n123 = Increment(x=w270) -> (x+1=w274:i32)
                n124 = Select(t=w274, s=w243, f=w270) -> (s? t:f=w269:i32)
                n125 = case shown="False" w243 {
                  tunnel: [w283 w287] -> w242
                  frame False {
                    w285 = T8[] [enum."S4 量測完成 產品NG_42"] items=["S2站PC動作中_20", "電流量測完成產品OK_21", "電流量測完成產品NG_22", "S2站Format 執行_23", "S2 Format OK_24", "S2 Format NG_25", "S2站燒入執行_26", "S2站燒入OK_27", "S2站燒入NG_28", "S2站動作完成_29", "S3 PC動作中_30", "S3 Format 此站執行_31", "S3 Format OK_32", "S3 Format NG_33", "S3 燒入程式 此站執行_34", "S3 燒入程式 OK_35", "S3 燒入程式 NG_36", "S3 備用_37", "S3 備用_38", "S3 動作完成_39", "S4 PC動作中_40", "S4 量測完成 產品正常_41", "S4 量測完成 產品NG_42", "S4 Format 此站執行_43", "S4 Format OK_44", "S4 Format NG_45", "S4 燒入 此站不執行_46", "S4 燒入程式 OK_47", "S4 燒入程式 NG_48", "S4 藍芽Scan OK_49", "S4 藍芽Scan NG_50", "S4 動作完成_51", "給PLC要量電流訊號", "給PLC要量電壓訊號"]
                    n126 = call "Set OutputPLC.vi"("Array"=w285, "Address In"=20) -> ("Error Out"=w283:errorcluster[])  [unwired: 9 in]
                  }
                  frame True {
                    w286 = T8[] [enum."S4 量測完成 產品正常_41"] items=["S2站PC動作中_20", "電流量測完成產品OK_21", "電流量測完成產品NG_22", "S2站Format 執行_23", "S2 Format OK_24", "S2 Format NG_25", "S2站燒入執行_26", "S2站燒入OK_27", "S2站燒入NG_28", "S2站動作完成_29", "S3 PC動作中_30", "S3 Format 此站執行_31", "S3 Format OK_32", "S3 Format NG_33", "S3 燒入程式 此站執行_34", "S3 燒入程式 OK_35", "S3 燒入程式 NG_36", "S3 備用_37", "S3 備用_38", "S3 動作完成_39", "S4 PC動作中_40", "S4 量測完成 產品正常_41", "S4 量測完成 產品NG_42", "S4 Format 此站執行_43", "S4 Format OK_44", "S4 Format NG_45", "S4 燒入 此站不執行_46", "S4 燒入程式 OK_47", "S4 燒入程式 NG_48", "S4 藍芽Scan OK_49", "S4 藍芽Scan NG_50", "S4 動作完成_51", "給PLC要量電流訊號", "給PLC要量電壓訊號"]
                    n127 = call "Set OutputPLC.vi"("Array"=w286, "Address In"=20) -> ("Error Out"=w287:errorcluster[])  [unwired: 9 in]
                  }
                }
                n128 = global read "Main Glb.vi" "Input Registers0-99"() -> (w252:u16[])
                n129 = Select(t="OK" ("DataIn"), s=w243, f="NG" ("DataIn")) -> (s? t:f=w244:string)
                n130 = call "Red PLC InReg.vi"("length"=10, "index"=10, "Input Registers Arr"=w252) -> ("Rad In Reg"=w251:string)  [unwired: 7 in, 1 out]
                n131 = call "Cub Meaasure FGV.vi"("Action"=Table_Save."Write" ("Enum"), 7:MeasureDisplayTab."Tray Barcode", "DataIn"=w244, "SN"=w251) -> ()  [unwired: 5 in, 7 out]
                n132 = Merge Errors(w242, w241) -> (w240:errorcluster)
              }
              frame "S2" {
                # "收尋S2站條碼"
                n133 = call "Retry Num.vi"("String"=w317) -> ("Numeric"=w332:i32, "retry次數"=w329:string[])  [unwired: 9 in]
                n134 = Index Array(array=w318, index=StationCmdSelect."Command") -> (element=w311:string)
                n135 = call "ToolScanTest.vi"("error in (no error)"=w319, "VISA resource name"=refnum<visa-resource-name> "COM10") -> ("error out"=w328:errorcluster, "read string 6"=w312:string)  [unwired: 4 in, 4 out]
                "Blue Scan2 receive" <- w312
                n136 = local write "retry次數"(w329) -> ()
                n137 = call "Tool RS232 test.vi"("error in (no error)"=w319, "Cmd In"=w311, "VISA resource name"=w293) -> ("error out"=w335:errorcluster, "receive string"=→"S2 receive":string)  [unwired: 7 in]
                n138 = call <vilib>:"Clear Errors.vi"("error in (no error)"=w328) -> ()  [unwired: 5 in, 2 out]
                n139 = local write "CurrentCmd"(w311) -> ()
                n140 = local write "Retry"(w332) -> ()
                n141 = Unbundle By Name(w335) -> ("status"=w324:bool)
                n142 = String Length(string=w312) -> (length=w327:i32)
                n143 = Not Equal To 0?(x=w327) -> (x != 0?=w326:bool)
                n144 = Not(x=w326) -> (.not. x?=w325:bool)
                n145 = Or(x=w325, y=w324) -> (x .or. y?=w323:bool)
                n146 = Not(x=w323) -> (.not. x?=w297:bool)
                n147 = call "Auto Inspection_Status.vi"("Action"=enum16{"Initial", "Write", "Read"}."Write", "DataIn"="SCAN2", "Station"=Auto_Inspection_Station_Name2."S2Measure", "Data"=Auto_Inspection_Data_Name."CurrentAction") -> ()  [unwired: 9 in, 3 out]
                n148 = Increment(x=w316) -> (x+1=w333:i32)
                n149 = Select(t=w333, s=w323, f=w316) -> (s? t:f=w330:i32)
                n150 = Increment(x=w320) -> (x+1=w334:i32)
                n151 = Greater Or Equal?(x=w330, y=w332) -> (x >= y?=w331:bool)
                n152 = Select(t=w334, s=w297, f=w320) -> (s? t:f=w313:i32)
                n153 = case shown="True" w331 {
                  tunnel: [errorcluster {"status"=FALSE, "code"=0, "source"=""} ("error constant") errorcluster {"status"=TRUE, "code"=11505, "source"=""} ("error constant")] -> w295
                  tunnel: w330 -> [w343 _]
                  tunnel: [w343 0] -> w315
                  frame False {
                  }
                  frame True {
                  }
                }
                n154 = case shown="False" w297 {
                  tunnel: [w337 w341] -> w296
                  frame False {
                    w339 = T8[] [enum."S4 量測完成 產品NG_42"] items=["S2站PC動作中_20", "電流量測完成產品OK_21", "電流量測完成產品NG_22", "S2站Format 執行_23", "S2 Format OK_24", "S2 Format NG_25", "S2站燒入執行_26", "S2站燒入OK_27", "S2站燒入NG_28", "S2站動作完成_29", "S3 PC動作中_30", "S3 Format 此站執行_31", "S3 Format OK_32", "S3 Format NG_33", "S3 燒入程式 此站執行_34", "S3 燒入程式 OK_35", "S3 燒入程式 NG_36", "S3 備用_37", "S3 備用_38", "S3 動作完成_39", "S4 PC動作中_40", "S4 量測完成 產品正常_41", "S4 量測完成 產品NG_42", "S4 Format 此站執行_43", "S4 Format OK_44", "S4 Format NG_45", "S4 燒入 此站不執行_46", "S4 燒入程式 OK_47", "S4 燒入程式 NG_48", "S4 藍芽Scan OK_49", "S4 藍芽Scan NG_50", "S4 動作完成_51", "給PLC要量電流訊號", "給PLC要量電壓訊號"]
                    n155 = call "Set OutputPLC.vi"("Array"=w339, "Address In"=20) -> ("Error Out"=w337:errorcluster[])  [unwired: 9 in]
                  }
                  frame True {
                    w340 = T8[] [enum."S4 量測完成 產品正常_41"] items=["S2站PC動作中_20", "電流量測完成產品OK_21", "電流量測完成產品NG_22", "S2站Format 執行_23", "S2 Format OK_24", "S2 Format NG_25", "S2站燒入執行_26", "S2站燒入OK_27", "S2站燒入NG_28", "S2站動作完成_29", "S3 PC動作中_30", "S3 Format 此站執行_31", "S3 Format OK_32", "S3 Format NG_33", "S3 燒入程式 此站執行_34", "S3 燒入程式 OK_35", "S3 燒入程式 NG_36", "S3 備用_37", "S3 備用_38", "S3 動作完成_39", "S4 PC動作中_40", "S4 量測完成 產品正常_41", "S4 量測完成 產品NG_42", "S4 Format 此站執行_43", "S4 Format OK_44", "S4 Format NG_45", "S4 燒入 此站不執行_46", "S4 燒入程式 OK_47", "S4 燒入程式 NG_48", "S4 藍芽Scan OK_49", "S4 藍芽Scan NG_50", "S4 動作完成_51", "給PLC要量電流訊號", "給PLC要量電壓訊號"]
                    n156 = call "Set OutputPLC.vi"("Array"=w340, "Address In"=20) -> ("Error Out"=w341:errorcluster[])  [unwired: 9 in]
                  }
                }
                n157 = Select(t="OK" ("DataIn"), s=w297, f="NG" ("DataIn")) -> (s? t:f=w298:string)
                n158 = global read "Main Glb.vi" "Input Registers0-99"() -> (w306:u16[])
                n159 = call "Red PLC InReg.vi"("length"=10, "index"=10, "Input Registers Arr"=w306) -> ("Rad In Reg"=w305:string)  [unwired: 7 in, 1 out]
                n160 = call "Cub Meaasure FGV.vi"("Action"=Table_Save."Write" ("Enum"), 7:MeasureDisplayTab."Tray Barcode", "DataIn"=w298, "SN"=w305) -> ()  [unwired: 5 in, 7 out]
                n161 = Merge Errors(w296, w295) -> (w294:errorcluster)
              }
              frame "D" {
                n162 = Index Array(array=w357, index=w354) -> (element=w356:dbl)
                n163 = Multiply(x=1000, y=w356) -> (x*y=w355:dbl)
                n164 = Wait (ms)(milliseconds to wait=w355) -> ()  [unwired: 1 out]
                n165 = call "Auto Inspection_Status.vi"("Action"=enum16{"Initial", "Write", "Read"}."Write", "DataIn"="Delay Time", "Station"=Auto_Inspection_Station_Name2."S2Measure", "Data"=Auto_Inspection_Data_Name."CurrentAction") -> ()  [unwired: 9 in, 3 out]
                n166 = Increment(x=w352) -> (x+1=w351:i32)
              }
              frame "T1" {
                (unwired) 10 ("index")
                w383 = u16 3 items=["SYSTem:VERSion?", "SYSTem:ERRor?", "*IDN?", "MEAS:CURR:DC?", "MEAS:VOLT?", "SYSTem:ERRor?"] ("Ringfor34450A")
                w382 = u16 5 items=["SYSTem:VERSion?", "SYSTem:ERRor?", "*IDN?", "MEAS:CURR:DC?", "MEAS:VOLT?", "MEAS:VOLT:DC?"] ("RingforIT8511")
                w380 = u16 1 items=["IT8511", "34450A", "WRBuff"] ("ChangeStatus")
                # "收尋S2站條碼"
                # "量電流"
                n167 = call "Retry Num.vi"("String"=w378) -> ("Numeric"=w389:i32, "retry次數"=w388:string[])  [unwired: 9 in]
                n168 = local write "retry次數"(w388) -> ()
                n169 = call "Auto Inspection_Status.vi"("Action"=enum16{"Initial", "Write", "Read"}."Write", "DataIn"="儀器34450A", "Station"=Auto_Inspection_Station_Name2."S2Measure", "Data"=Auto_Inspection_Data_Name."CurrentAction") -> ()  [unwired: 9 in, 3 out]
                n170 = local write "Retry"(w389) -> ()
                n171 = call "MTool34450A.vi"("Ringfor34450A"=w383, "RingforIT8511"=w382, "VISA resource name"=refnum<visa-resource-name> "USB0::0x2A8D::0xB318::MY59430005::INSTR", "ChangeStatus"=w380) -> ("error out"=w384:errorcluster, 1:"μA"=w363:string, 2:"μA"=→"T1 μA":dbl, "read buffer"=→"T1 buffer":string)  [unwired: 4 in]
                n172 = Unbundle By Name(w384) -> ("status"=w386:bool)
                n173 = Increment(x=w379) -> (x+1=w390:i32)
                n174 = Select(t=w390, s=w386, f=w379) -> (s? t:f=w387:i32)
                n175 = Not(x=w386) -> (.not. x?=w362:bool)
                n176 = Greater Or Equal?(x=w387, y=w389) -> (x >= y?=w385:bool)
                n177 = Increment(x=w377) -> (x+1=w391:i32)
                n178 = Select(t=w391, s=w362, f=w377) -> (s? t:f=w376:i32)
                n179 = case shown="False" w385 {
                  tunnel: [errorcluster {"status"=FALSE, "code"=0, "source"=""} ("error constant") w403] -> w360
                  tunnel: w387 -> [w401 _]
                  tunnel: [w401 0] -> w375
                  tunnel: w384 -> [_ w403]
                  frame False {
                  }
                  frame True {
                  }
                }
                n180 = Select(t=w363, s=w362, f="NG" ("DataIn")) -> (s? t:f=w364:string)
                n181 = global read "Main Glb.vi" "Input Registers0-99"() -> (w370:u16[])
                n182 = case shown="False" w362 {
                  tunnel: [w395 w398] -> w361
                  frame False {
                    w397 = T8[] [enum."電流量測完成產品NG_22"] items=["S2站PC動作中_20", "電流量測完成產品OK_21", "電流量測完成產品NG_22", "S2站Format 執行_23", "S2 Format OK_24", "S2 Format NG_25", "S2站燒入執行_26", "S2站燒入OK_27", "S2站燒入NG_28", "S2站動作完成_29", "S3 PC動作中_30", "S3 Format 此站執行_31", "S3 Format OK_32", "S3 Format NG_33", "S3 燒入程式 此站執行_34", "S3 燒入程式 OK_35", "S3 燒入程式 NG_36", "S3 備用_37", "S3 備用_38", "S3 動作完成_39", "S4 PC動作中_40", "S4 量測完成 產品正常_41", "S4 量測完成 產品NG_42", "S4 Format 此站執行_43", "S4 Format OK_44", "S4 Format NG_45", "S4 燒入 此站不執行_46", "S4 燒入程式 OK_47", "S4 燒入程式 NG_48", "S4 藍芽Scan OK_49", "S4 藍芽Scan NG_50", "S4 動作完成_51", "給PLC要量電流訊號", "給PLC要量電壓訊號"]
                    n183 = call "Set OutputPLC.vi"("Array"=w397, "Address In"=20) -> ("Error Out"=w395:errorcluster[])  [unwired: 9 in]
                  }
                  frame True {
                    w399 = T8[] [enum."電流量測完成產品OK_21"] items=["S2站PC動作中_20", "電流量測完成產品OK_21", "電流量測完成產品NG_22", "S2站Format 執行_23", "S2 Format OK_24", "S2 Format NG_25", "S2站燒入執行_26", "S2站燒入OK_27", "S2站燒入NG_28", "S2站動作完成_29", "S3 PC動作中_30", "S3 Format 此站執行_31", "S3 Format OK_32", "S3 Format NG_33", "S3 燒入程式 此站執行_34", "S3 燒入程式 OK_35", "S3 燒入程式 NG_36", "S3 備用_37", "S3 備用_38", "S3 動作完成_39", "S4 PC動作中_40", "S4 量測完成 產品正常_41", "S4 量測完成 產品NG_42", "S4 Format 此站執行_43", "S4 Format OK_44", "S4 Format NG_45", "S4 燒入 此站不執行_46", "S4 燒入程式 OK_47", "S4 燒入程式 NG_48", "S4 藍芽Scan OK_49", "S4 藍芽Scan NG_50", "S4 動作完成_51", "給PLC要量電流訊號", "給PLC要量電壓訊號"]
                    n184 = call "Set OutputPLC.vi"("Array"=w399, "Address In"=20) -> ("Error Out"=w398:errorcluster[])  [unwired: 9 in]
                  }
                }
                n185 = call "Red PLC InReg.vi"("length"=10, "Input Registers Arr"=w370) -> ("Rad In Reg"=w369:string)  [unwired: 8 in, 1 out]
                n186 = call "Cub Meaasure FGV.vi"("Action"=Table_Save."Write" ("Enum"), 7:MeasureDisplayTab."Tray Barcode", "DataIn"=w364, "SN"=w369) -> ()  [unwired: 5 in, 7 out]
                n187 = Merge Errors(w361, w360) -> (w359:errorcluster)
              }
              frame "T2" {
                w432 = u16 3 items=["SYSTem:VERSion?", "SYSTem:ERRor?", "*IDN?", "MEAS:CURR:DC?", "MEAS:VOLT?", "SYSTem:ERRor?"] ("Ringfor34450A")
                w431 = u16 5 items=["SYSTem:VERSion?", "SYSTem:ERRor?", "*IDN?", "MEAS:CURR:DC?", "MEAS:VOLT?", "MEAS:VOLT:DC?"] ("RingforIT8511")
                w429 = u16 0 items=["IT8511", "34450A", "WRBuff"] ("ChangeStatus")
                # "收尋S2站條碼"
                # "量電壓"
                n188 = call "Auto Inspection_Status.vi"("Action"=enum16{"Initial", "Write", "Read"}."Write", "DataIn"="IT8511", "Station"=Auto_Inspection_Station_Name2."S2Measure", "Data"=Auto_Inspection_Data_Name."CurrentAction") -> ()  [unwired: 9 in, 3 out]
                n189 = call "Retry Num.vi"("String"=w423) -> ("Numeric"=w438:i32, "retry次數"=w437:string[])  [unwired: 9 in]
                n190 = local write "retry次數"(w437) -> ()
                n191 = local write "Retry"(w438) -> ()
                n192 = call "MTool34450A.vi"("Ringfor34450A"=w432, "RingforIT8511"=w431, "VISA resource name"=refnum<visa-resource-name> "COM11", "ChangeStatus"=w429) -> ("error out"=w434:errorcluster, "μA"=→"T2 μA":dbl, "read buffer"=w410:string)  [unwired: 4 in, 1 out]
                "T2 buffer" <- w410
                n193 = Unbundle By Name(w434) -> ("status"=w408:bool)
                n194 = Increment(x=w424) -> (x+1=w433:i32)
                n195 = Not(x=w408) -> (.not. x?=w409:bool)
                n196 = Select(t=w433, s=w408, f=w433) -> (s? t:f=w436:i32)
                n197 = Greater Or Equal?(x=w436, y=w438) -> (x >= y?=w435:bool)
                n198 = Increment(x=w425) -> (x+1=w439:i32)
                n199 = Select(t=w410, s=w409, f="NG" ("DataIn")) -> (s? t:f=w411:string)
                n200 = global read "Main Glb.vi" "Input Registers0-99"() -> (w418:u16[])
                n201 = Select(t=w439, s=w409, f=w425) -> (s? t:f=w426:i32)
                n202 = case shown="False" w435 {
                  tunnel: [errorcluster {"status"=FALSE, "code"=0, "source"=""} ("error constant") w449] -> w406
                  tunnel: w436 -> [w447 _]
                  tunnel: [w447 0] -> w428
                  tunnel: w434 -> [_ w449]
                  frame False {
                  }
                  frame True {
                  }
                }
                n203 = case shown="True" w408 {
                  tunnel: [w441 w444] -> w407
                  frame False {
                    w443 = T8[] [enum."S4 量測完成 產品NG_42"] items=["S2站PC動作中_20", "電流量測完成產品OK_21", "電流量測完成產品NG_22", "S2站Format 執行_23", "S2 Format OK_24", "S2 Format NG_25", "S2站燒入執行_26", "S2站燒入OK_27", "S2站燒入NG_28", "S2站動作完成_29", "S3 PC動作中_30", "S3 Format 此站執行_31", "S3 Format OK_32", "S3 Format NG_33", "S3 燒入程式 此站執行_34", "S3 燒入程式 OK_35", "S3 燒入程式 NG_36", "S3 備用_37", "S3 備用_38", "S3 動作完成_39", "S4 PC動作中_40", "S4 量測完成 產品正常_41", "S4 量測完成 產品NG_42", "S4 Format 此站執行_43", "S4 Format OK_44", "S4 Format NG_45", "S4 燒入 此站不執行_46", "S4 燒入程式 OK_47", "S4 燒入程式 NG_48", "S4 藍芽Scan OK_49", "S4 藍芽Scan NG_50", "S4 動作完成_51", "給PLC要量電流訊號", "給PLC要量電壓訊號"]
                    n204 = call "Set OutputPLC.vi"("Array"=w443, "Address In"=20) -> ("Error Out"=w441:errorcluster[])  [unwired: 9 in]
                  }
                  frame True {
                    w445 = T8[] [enum."S4 量測完成 產品正常_41"] items=["S2站PC動作中_20", "電流量測完成產品OK_21", "電流量測完成產品NG_22", "S2站Format 執行_23", "S2 Format OK_24", "S2 Format NG_25", "S2站燒入執行_26", "S2站燒入OK_27", "S2站燒入NG_28", "S2站動作完成_29", "S3 PC動作中_30", "S3 Format 此站執行_31", "S3 Format OK_32", "S3 Format NG_33", "S3 燒入程式 此站執行_34", "S3 燒入程式 OK_35", "S3 燒入程式 NG_36", "S3 備用_37", "S3 備用_38", "S3 動作完成_39", "S4 PC動作中_40", "S4 量測完成 產品正常_41", "S4 量測完成 產品NG_42", "S4 Format 此站執行_43", "S4 Format OK_44", "S4 Format NG_45", "S4 燒入 此站不執行_46", "S4 燒入程式 OK_47", "S4 燒入程式 NG_48", "S4 藍芽Scan OK_49", "S4 藍芽Scan NG_50", "S4 動作完成_51", "給PLC要量電流訊號", "給PLC要量電壓訊號"]
                    n205 = call "Set OutputPLC.vi"("Array"=w445, "Address In"=20) -> ("Error Out"=w444:errorcluster[])  [unwired: 9 in]
                  }
                }
                n206 = call "Red PLC InReg.vi"("length"=10, "index"=10, "Input Registers Arr"=w418) -> ("Rad In Reg"=w417:string)  [unwired: 7 in, 1 out]
                n207 = call "Cub Meaasure FGV.vi"("Action"=Table_Save."Write" ("Enum"), 7:MeasureDisplayTab."Tray Barcode", "DataIn"=w411, "SN"=w417) -> ()  [unwired: 5 in, 7 out]
                n208 = Merge Errors(w407, w406) -> (w405:errorcluster)
              }
            }
          }
          frame True {
            w451 = TRUE
            "Boolean" <- w451
          }
        }
        n209 = property class="DigNum (strict)"(reference=w64, "Value"=w63) -> ()  [unwired: 1 in, 2 out]
        n210 = Compound Arithmetic op=OR(w61, w68, "stop") -> (w67:bool)
      }
    }
    frame Enabled {
    }
  }
  n211 = disable-structure shown="Disabled" {
    frame Disabled {
      n212 = while {
        tunnel: cluster{"Table Control":string[][]}[] [{"Table Control"=[]}] ("Array 2") -> [w459]
        shift-right: [w458] -> w452
        shift-left: _ -> [w456]
        stop <- TRUE stop-if-true
        n213 = case shown="\"Add\"" "Enum" {
          tunnel: w459 -> [w461 _ _ _ _ _]
          tunnel: [w461 w465 w470 w495 w517 w524] -> w458
          tunnel: "Table Control 3" -> [_ w463 w472 w486 _ _]
          tunnel: w456 -> [_ w462 w467 w493 w516 w524]
          tunnel: "SN" -> [_ _ w466 w492 w515 _]
          frame "initial", Default {
          }
          frame "Add" {
            n214 = Bundle("Table Control 3"=w463) -> (w464:cluster{"Table Control 3":string[][]})  [unwired: 1 in]
            n215 = Build Array (concatenate)(w462, w464) -> (w465:cluster{"Table Control 3":string[][]}[])
            n216 = Bundle() -> ()  [unwired: 2 in, 1 out]
          }
          frame "Write" {
            n217 = for {
              tunnel: w467 -> [w480] mode=indexing
              tunnel: [w476] -> w475 mode=indexing
              n218 = Unbundle By Name(w480) -> ("Table Control 3"=w479:string[][])
              n219 = Index Array(array=w479, index (row)=0 ("disabled index (col)"), index (col)=1 ("disabled index (col)")) -> (element=w476:string)
            }
            n220 = Search 1D Array(1D array=w475, element=w466) -> (index of element=w471:i32)  [unwired: 1 in]
            n221 = Index Array(array=w467, index=w471) -> (element=w474:cluster{"Table Control 3":string[][]})
            n222 = Unbundle By Name(w474) -> ("Table Control 3"=w473:string[][])
            n223 = Build Array (concatenate)(w473, w472) -> (w469:string[][])
            n224 = Bundle(w469) -> (w468:cluster{string[][]})  [unwired: 1 in]
            n225 = Replace Array Subset(array=w467, new element=w468, index=w471) -> (w470:cluster{"Table Control 3":string[][]}[])
          }
          frame "Replace" {
            n226 = for {
              tunnel: w493 -> [w509] mode=indexing
              tunnel: [w505] -> w497 mode=indexing
              n227 = Unbundle By Name(w509) -> ("Table Control 3"=w508:string[][])
              n228 = Index Array(array=w508, index (row)=0 ("disabled index (col)"), index (col)=1 ("disabled index (col)")) -> (element=w505:string)
            }
            n229 = Search 1D Array(1D array=w497, element=w492) -> (index of element=w490:i32)  [unwired: 1 in]
            n230 = Index Array(array=w493, index=w490) -> (element=w496:cluster{"Table Control 3":string[][]})
            n231 = Unbundle By Name(w496) -> ("Table Control 3"=w483:string[][])
            n232 = Array Size(array=w486) -> (size(s)=w488:i32[])
            n233 = Index Array(array=w486, index (col)=1 ("disabled index (col)")) -> (element=w484:string[])  [unwired: 1 in]
            n234 = Index Array(array=w488) -> (element #1=w487:i32)  [unwired: 2 in, 1 out]
            n235 = Array Size(array=w483) -> (size(s)=w489:i32[])
            n236 = Index Array(array=w489) -> (element #1=w482:i32)  [unwired: 2 in, 1 out]
            n237 = Subtract(x=w482, y=w487) -> (x-y=w481:i32)
            n238 = for {
              shift-right: [w504] -> w491
              shift-left: w483 -> [w503]
              tunnel: w481 -> [w500]
              tunnel: w484 -> [w499] mode=indexing
              i -> [w501]
              n239 = Add(x=w500, y=w501) -> (x+y=w498:i32)
              n240 = Replace Array Subset(array=w503, new element=w499, index (row)=w498, index (col)=1 ("disabled index (col)")) -> (w504:string[][])
            }
            n241 = Bundle("Table Control 3"=w491) -> (w494:cluster{"Table Control 3":string[][]})  [unwired: 1 in]
            n242 = Replace Array Subset(array=w493, new element=w494, index=w490) -> (w495:cluster{"Table Control 3":string[][]}[])
          }
          frame "Delete" {
            n243 = for {
              tunnel: w516 -> [w523] mode=indexing
              tunnel: [w519] -> w518 mode=indexing
              n244 = Unbundle By Name(w523) -> ("Table Control 3"=w522:string[][])
              n245 = Index Array(array=w522, index (row)=0 ("disabled index (col)"), index (col)=1 ("disabled index (col)")) -> (element=w519:string)
            }
            n246 = Search 1D Array(1D array=w518, element=w515) -> (index of element=w514:i32)  [unwired: 1 in]
            n247 = Index Array(array=w516, index=w514) -> ()  [unwired: 1 out]
            n248 = Delete From Array(array=w516, length=1, index=w514) -> (deleted portion=w512:cluster{"Table Control 3":string[][]}[], array with subset deleted=w517:cluster{"Table Control 3":string[][]}[])
            n249 = Index Array(array=w512) -> (element=w511:cluster{"Table Control 3":string[][]})  [unwired: 1 in]
            n250 = Unbundle By Name(w511) -> ("Table Control 3"=→"LOG":string[][])
          }
          frame "REad" {
          }
        }
      }
      "Array 3" <- w452
    }
    frame Enabled {
    }
  }
  n251 = disable-structure shown="Disabled" {
    frame Disabled {
      n252 = call "Save Table Test.vi"() -> ()  [unwired: 10 in, 2 out]
    }
    frame Enabled {
    }
  }
